vi "Generate write queue item.vi"(8 "error in (no error)":errorcluster, 9 "Subscription ID":u64, 10 "Request ID":u64, 11 "IUnsubscribe in":refnum<class "IUnsubscribe.lvclass">) -> (0 "error out":errorcluster, 2 "Write queue item":T1, 3 "IUnsubscribe out":refnum<class "IUnsubscribe.lvclass">)   [LabVIEW 2020, in "wamplv.lvlib" / "IUnsubscribe.lvclass"]
uses:
  IUnsubscribe.lvclass
  TypeDefs/Transport type.ctl
  wamplv.lvlib
  WAMP Client/Private/TypeDef/Write queue item.ctl
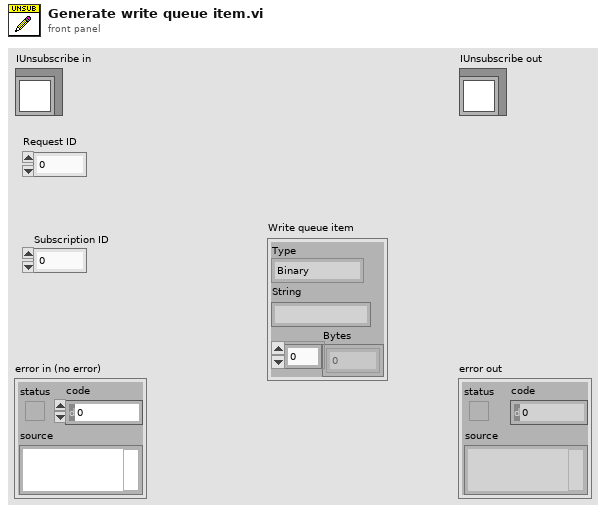
[diagram p1: front panel]
types:
  T1 = typedef "wamplv.lvlib/Write queue item.ctl" = cluster{"Type":T2, "String":string, "Bytes":u8[]}
  T2 = typedef "wamplv.lvlib/Transport type.ctl" = enum16{"Binary", "Text"}
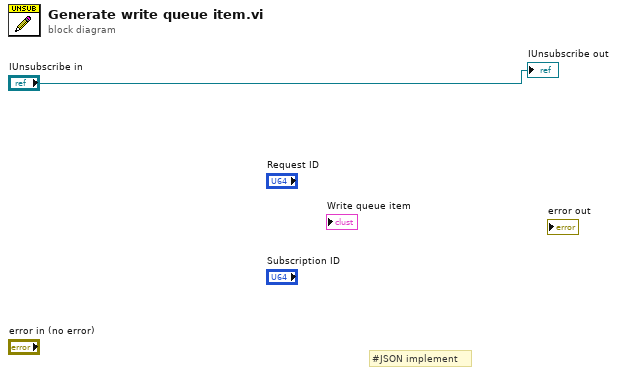
[diagram p0: block diagram]
diagram:
  # "#JSON implement"
  "IUnsubscribe out" <- "IUnsubscribe in"
